vi "Acquisition Example.vi"() -> ()   [LabVIEW 2023, in "GettingStarted_Acq_148X_Host.lvlib"]
uses:
  GettingStarted_Acq_148X_Host.lvlib
  <vilib>/rvi/interface/nirviCloseFPGA/nirviCloseFPGA.xnode
  <instrlib>/FlexRIO/API/Host/v1/NI FlexRIO API v1.lvlib
  Common/GettingStarted_Common_148X_Host.lvlib
  <vilib>/vision/Image Controls.llb/IMAQ Image.ctl
  Common/Types/Packet Table.ctl
  <vilib>/Utility/miscctls.llb/LVRowAndColumnUnsignedTypeDef.ctl
  <vilib>/FPGAPlugInAG/Dynamic/niLvFpga_Close_Dynamic.vi
  <instrlib>/FlexRIO/API/Host/v1/NI FlexRIO/API/Wait for PoC Safe to Disconnect Channels Array.vi
  <instrlib>/FlexRIO/CSI-2/v2/Common/Types/LLP Data Type.ctl
  <instrlib>/FlexRIO/CSI-2/v2/Common/NI CSI-2 API Common v2.lvlib
  <vilib>/userDefined/Silver/nirio_resource_slv.ctl
  Types/CSI-2 Data Source.ctl
  Common/Types/Serial Channel Configuration.ctl
  Common/Types/RAW Interpretation for Display.ctl
  <instrlib>/FlexRIO/CSI-2/v2/FPGA/Types/Timestamp ID.ctl
  <instrlib>/FlexRIO/CSI-2/v2/FPGA/NI CSI-2 API FPGA v2.lvlib
  Common/Types/GPIO Filter.ctl
  FPGA/Common/Types/SerDes Identifier.ctl
  FPGA/Common/GettingStarted_Common_148X_FPGA.lvlib
  <instrlib>/FlexRIO/CSI-2/v2/FPGA/Types/GPIO Bank.ctl
  <instrlib>/FlexRIO/CSI-2/v2/FPGA/Types/Display Parameters.ctl
panel:
  out "Acquisition Stopped":bool
  in  "Configuration":T1(tab)
  in  "Logged Packets to Display":i64=1400
  in  "Log Packets to Disk":bool
  in  "Bitfile Path":path
  in  "TDMS File Directory":path
  in  "RIO Device":T2
  in  "Display Acquired Images":bool=TRUE
  in  "Log I2C to Disk":bool
  in  "Log GPIO to Disk":bool
  in  "Channel Configurations":T3[](array[typedef])=[{"Serial Channel"="SI0", "FPGA Display Parameters"={"virtual channel"=0.0, "payload data type"=enum."RAW 12", "frame skip count"=0, "line skip count"=0, "pixel skip count"=0.0}, "RAW Display Parameters"={"Interpretation"=enum."Bayer", "Bayer Parameters"={"Pattern"=3, "Algorithm"=0, "Red Gain"=1.0, "Green Gain"=1.0, "Blue Gain"=1.0}}}] {"RAW Display Parameters"."Bayer Parameters"."Blue Gain" min=0.0 max=3.99 step=0.1 format="%_4g"; "RAW Display Parameters"."Bayer Parameters"."Green Gain" min=0.0 max=3.99 step=0.1 format="%_4g"; "RAW Display Parameters"."Bayer Parameters"."Red Gain" min=0.0 max=3.99 step=0.1 format="%_4g"; "RAW Display Parameters"."Bayer Parameters"."Algorithm" items=["Bilinear", "VNG"]; "RAW Display Parameters"."Bayer Parameters"."Pattern" items=["GB", "GR", "BG", "RG"]}
  in  "CSI-2 Data Source":T7=1 items=["Raw", "Corrected"]
  in  "Configuration Script":path
  in  "Acquisition Duration (s)":dbl=1.0 format="%#_13g"
  in  "Continuous Acquisition":bool=TRUE
  in  "Data Type Filter":T5[](array[typedef])
  in  "Virtual Channel Filter":fxp<+,4,4>[](array[numeric])
  in  "Invert Data Type Filter":bool
  in  "Invert Virtual Channel Filter":bool
  in  "Enable First and Last Packet Select":bool=TRUE
  in  "Stop Timeout (s)":dbl=1.0
  in  "First Packet Data Type Select":T5
  in  "Last Packet Data Type Select":T5=enum."Frame End"
  in  "Serial Input Active Lane Count":i32(ring)=4 items=["1 Lane"=1, "2 Lanes"=2, "4 Lanes"=4]
  in  "Reference Clock Frequency (Hz)":dbl=25000000.0 format="%#_6p"
  in  "Power Over Coax Source":i32(ring) items=["None", "Internal", "Auxiliary"]
  in  "timestamp filter":T8[](array[typedef])
  in  "GPIO to Display":T9[](array[typedef])
  in  "GPIO Bank Select":T10
  in  "Write GPIO":bool
  in  "GPIO Bank Write":T11
  out "GPIO Bank Read":T11
  out "Acquisition Duration (s)":dbl format="%.1f"
  out "Acquisition In Progress":bool
  out "Power Over Coax Voltage (V)":dbl[](array[numeric]) format="%#.2pV"
  out "Power Over Coax Current (A)":dbl[](array[numeric]) format="%#.2pA"
  in  "Acquired Serial Input Channel Data":T12(tab)
  out "Source Rate (fps)(1st Display)":dbl
  out "Update Rate (fps)(1st Display)":dbl
  in  "Serial Channel (1st Display)":fxp<+,3,3>
  out "1st channel display":T13(plugin-control)
  out "Source Rate (fps)(2nd Display)":dbl
  out "Update Rate (fps)(2nd Display)":dbl
  out "2nd channel display":T13(plugin-control)
  in  "Serial Channel (2nd Display)":fxp<+,3,3>
  out "Bytes Acquired (1st Channel)":i64 format="%#.6p"
  out "Acquired Packets (1st Channel)":T14
  out "Packets Logged (1st Channel)":i64
  out "Bytes Acquired (2nd Channel)":i64 format="%#.6p"
  out "Acquired Packets (2nd Channel)":T14
  out "Packets Logged (2nd Channel)":i64
  out "I2C Timestamps":T14
  out "GPIO Timestamps Waveform":digitalwaveform[](graph)
  out "Error Parsing GPIO Timestamps":bool
  out "Power Over Coax Source In Range":bool[](array[boolean])
  in  "Stop Acquisition":bool
  out "Error Out":errorcluster
  # "Overview: Configure an acquisition for a CSI-2 sensor and transfer the acquired data and timestamps to disk.  \nInstructions: Visit https://ni.com/r/automotive-camera-module-ref for tutorials and reference material on using this example with the PXIe-148X."
  # "Configuration Settings"
  # "Data Output"
  # "Resource Configuration"
  # "Data Output Configuration"
  # "Channel Configuration"
  # "Acquisition Configuration"
  # "First and Last Packet Select Configuration"
  # "Packet Filter Configuration"
  # "Power Over Coax Configuration"
  # "Clocking Configuration"
  # "I2C Timestamp Configuration"
  # "The timestamp filters listed correspond to the I2C traffic for a specific serial channel:\n\nUser24 = SI0\nUser25 = SI1\nUser26 = SI2\nUser27 = SI3\nUser28 = SI4\nUser29 = SI5\nUser30 = SI6\nUser31 = SI7"
  # "GPIO Configuration"
  # "* For additional packet viewing capability, use GettingStarted_Common_148X_Host.lvlib->TDMS File Viewer.vi"
  # "* For additional packet viewing capability, use GettingStarted_Common_148X_Host.lvlib->TDMS File Viewer.vi"
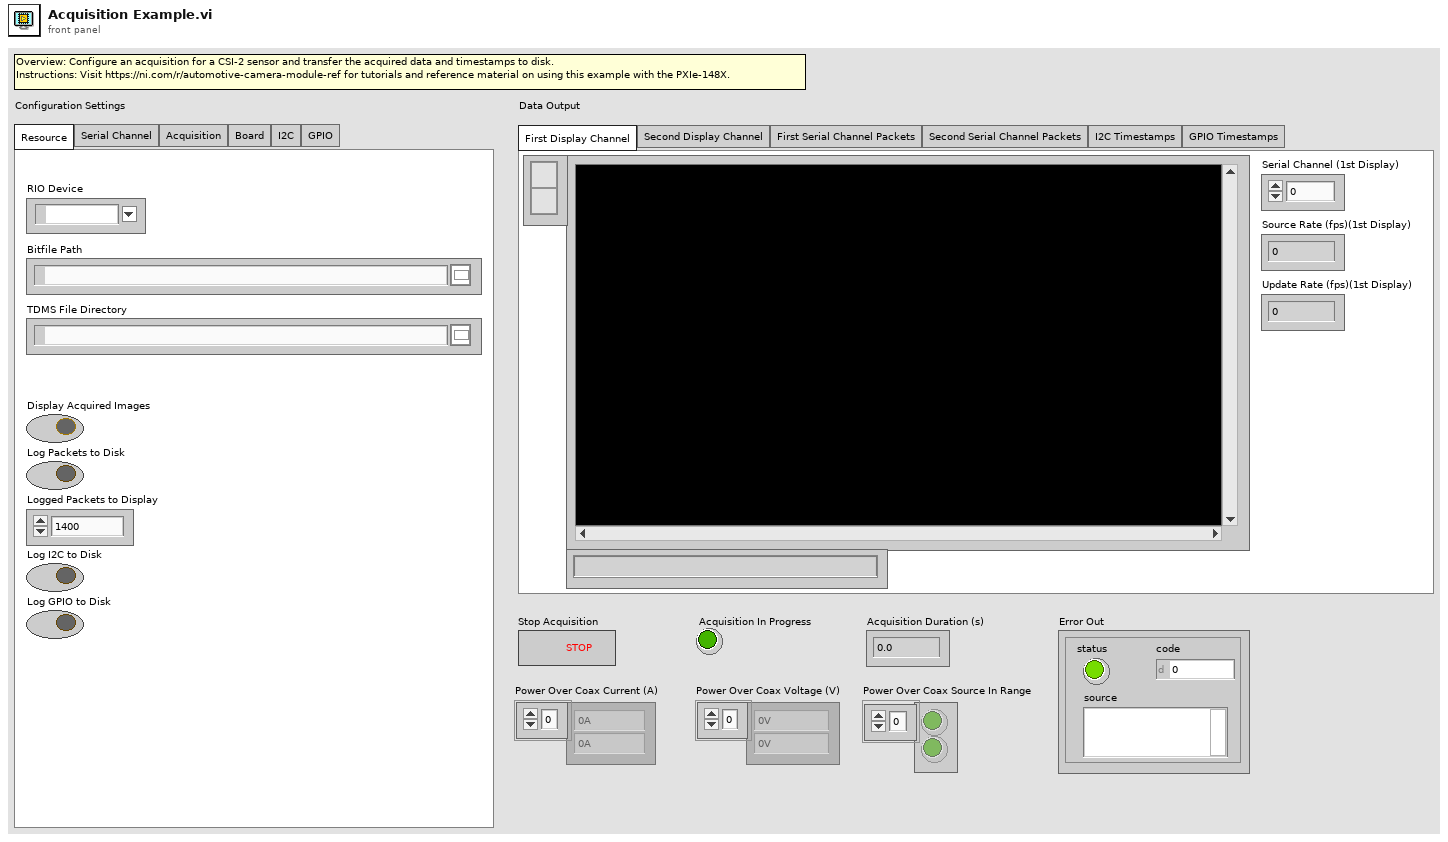
[diagram p1: front panel]
types:
  T1 = enum32{"Resource", "Serial Channel", "Acquisition", "Board", "I2C", "GPIO"}
  T2 = typedef "nirio_resource_slv.ctl" = tag
  T3 = typedef "GettingStarted_Common_148X_Host.lvlib/Serial Channel Configuration.ctl" = cluster{"Serial Channel":string, "FPGA Display Parameters":T4, "RAW Display Parameters":cluster{"Interpretation":T6, "Bayer Parameters":cluster{"Pattern":i32, "Algorithm":i32, "Red Gain":dbl, "Green Gain":dbl, "Blue Gain":dbl}}}
  T4 = typedef "NI CSI-2 API FPGA v2.lvlib/Display Parameters.ctl" = cluster{"virtual channel":fxp<+,4,4>, "payload data type":T5, "frame skip count":u16, "line skip count":u8, "pixel skip count":fxp<+,5,5>}
  T5 = typedef "NI CSI-2 API Common v2.lvlib/LLP Data Type.ctl" = enum8{"Frame Start", "Frame End", "Line Start", "Line End", "End of Transmission", "Reserved 0", "Reserved 1", "Reserved 2", "Generic Short Packet 1", "Generic Short Packet 2", "Generic Short Packet 3", "Generic Short Packet 4", "Generic Short Packet 5", "Generic Short Packet 6", "Generic Short Packet 7", "Generic Short Packet 8", "Null", "Blanking Data", "Embedded 8-bit non Image Data", "Generic Long Packet 1", "Generic Long Packet 2", "Generic Long Packet 3", "Generic Long Packet 4", "Reserved 3", "YUV420 8-bit", "YUV420 10-bit", "Legacy YUV420 8-bit", "Reserved 4", "YUV420 8-bit Chroma Shifted", "YUV420 10-bit Chroma Shifted", "YUV422 8-bit", "YUV422 10-bit", "RGB444", "RGB555", "RGB565", "RGB666", "RGB888", "Reserved 5", "Reserved 6", "RAW 24", "RAW 6", "RAW 7", "RAW 8", "RAW 10", "RAW 12", "RAW 14", "RAW 16", "RAW 20", "User Defined 8-bit Data 1", "User Defined 8-bit Data 2", "User Defined 8-bit Data 3", "User Defined 8-bit Data 4", "User Defined 8-bit Data 5", "User Defined 8-bit Data 6", "User Defined 8-bit Data 7", "User Defined 8-bit Data 8", "USL Command", "Reserved 7", "Reserved 8", "Reserved 9", "Reserved 10", "Reserved 11", "Reserved 12", "LRTE EPD Spacer"}
  T6 = typedef "GettingStarted_Common_148X_Host.lvlib/RAW Interpretation for Display.ctl" = enum16{"Grayscale", "Bayer", "RGB", "YUV422", "YUV420", "Legacy YUV420"}
  T7 = typedef "GettingStarted_Acq_148X_Host.lvlib/CSI-2 Data Source.ctl" = u16
  T8 = typedef "NI CSI-2 API FPGA v2.lvlib/Timestamp ID.ctl" = enum8{"SI0 LLP", "SI1 LLP", "SI2 LLP", "SI3 LLP", "SI4 LLP", "SI5 LLP", "SI6 LLP", "SI7 LLP", "SO0 LLP", "SO1 LLP", "SO2 LLP", "SO3 LLP", "SO4 LLP", "SO5 LLP", "SO6 LLP", "SO7 LLP", "Ser0 GPIO Bank", "Ser1 GPIO Bank", "Ser2 GPIO Bank", "Ser3 GPIO Bank", "Ser4 GPIO Bank", "Ser5 GPIO Bank", "Ser6 GPIO Bank", "Ser7 GPIO Bank", "Des0 GPIO Bank", "Des1 GPIO Bank", "Des2 GPIO Bank", "Des3 GPIO Bank", "Des4 GPIO Bank", "Des5 GPIO Bank", "Des6 GPIO Bank", "Des7 GPIO Bank", "User0", "User1", "User2", "User3", "User4", "User5", "User6", "User7", "User8", "User9", "User10", "User11", "User12", "User13", "User14", "User15", "User16", "User17", "User18", "User19", "User20", "User21", "User22", "User23", "User24", "User25", "User26", "User27", "User28", "User29", "User30", "User31"}
  T9 = typedef "GettingStarted_Common_148X_Host.lvlib/GPIO Filter.ctl" = cluster{"GPIO Bank":T8, "GPIO Number":i32}
  T10 = typedef "GettingStarted_Common_148X_FPGA.lvlib/SerDes Identifier.ctl" = enum8{"None", "SI 0 Deserializer", "SI 1 Deserializer", "SI 2 Deserializer", "SI 3 Deserializer", "SI 4 Deserializer", "SI 5 Deserializer", "SI 6 Deserializer", "SI 7 Deserializer", "SO 0 Serializer", "SO 1 Serializer", "SO 2 Serializer", "SO 3 Serializer", "SO 4 Serializer", "SO 5 Serializer", "SO 6 Serializer", "SO 7 Serializer", "SI 0 SI 1 Deserializer", "SI 2 SI 3 Deserializer", "SI 4 SI 5 Deserializer", "SI 6 SI 7 Deserializer"}
  T11 = typedef "NI CSI-2 API FPGA v2.lvlib/GPIO Bank.ctl" = cluster{"GPIO 0":bool, "GPIO 1":bool, "GPIO 2":bool, "GPIO 3":bool, "GPIO 4":bool, "GPIO 5":bool, "GPIO 6":bool, "GPIO 7":bool, "GPIO 8":bool, "GPIO 9":bool, "GPIO 10":bool}
  T12 = enum32{"First Display Channel", "Second Display Channel", "First Serial Channel Packets", "Second Serial Channel Packets", "I2C Timestamps", "GPIO Timestamps"}
  T13 = typedef "IMAQ Image.ctl" = refnum<image>
  T14 = typedef "GettingStarted_Common_148X_Host.lvlib/Packet Table.ctl" = string[][]
  T15 = typedef "LVRowAndColumnUnsignedTypeDef.ctl" = cluster{"Row":u32, "Column":u32}
  T16 = typedef "GettingStarted_Common_148X_Host.lvlib/Serial Channel Display Parameters.ctl" = cluster{"images":cluster{"grayscale":T13, "color":T13}, "RAW parameters":cluster{"interpretation":T6, "bayer parameters":cluster{"pattern":i32, "algorithm":i32, "red gain":dbl, "green gain":dbl, "blue gain":dbl}}}
  T17 = cluster{"Source Rate (fps)(1st Display)":refnum<vi>, "Update Rate (fps)(1st Display)":refnum<vi>}
  T18 = cluster{"Source Rate (fps)(2nd Display)":refnum<vi>, "Update Rate (fps)(2nd Display)":refnum<vi>}
  T19 = cluster{"Source Rate (fps)(2nd Display)":refnum<vi>, "Update Rate (fps)(2nd Display)":refnum<vi>}[]
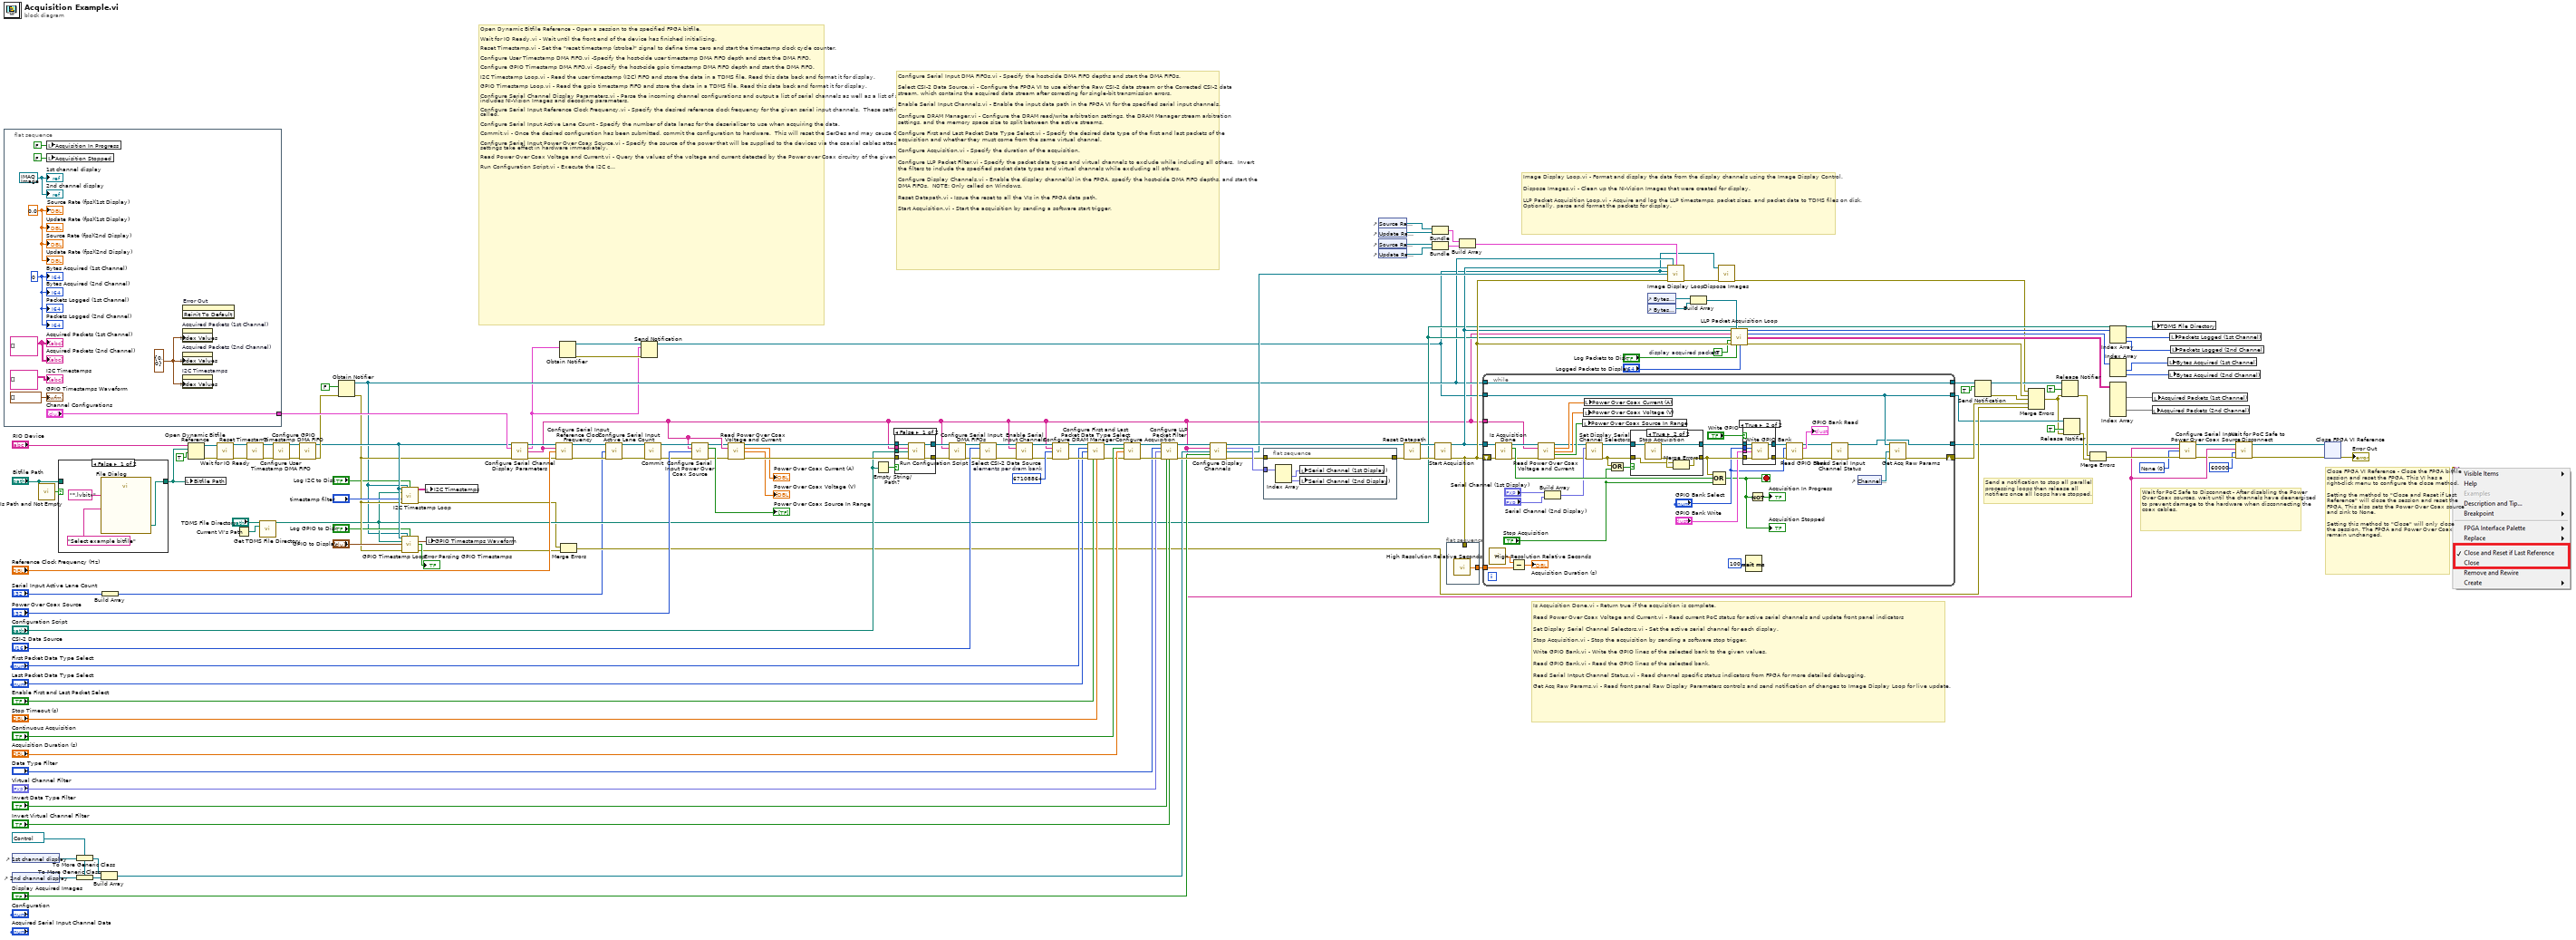
[diagram p0: block diagram]
diagram:
  w4 = 0 items=["None", "Internal", "Auxiliary"] ("power over coax source")
  w31 = TRUE  # display acquired packets
  w82 = refnum<vi> refnum ("image display reference")
  w148 = u32 67108864  # elements per dram bank
  # "Wait for PoC Safe to Disconnect - After disabling the Power Over Coax sources, wait until the channels have deenergized to prevent damage to the hardware when disconnecting the coax cables."
  # "Send a notification to stop all parallel processing loops then release all notifiers once all loops have stopped."
  # "Image Display Loop.vi - Format and display the data from the display channels using the Image Display Control.   \n\nDispose Images.vi - Clean up the NI-Vision Images that were created for display.\n\nLLP Packet Acquisition Loop.vi - Acquire and log the LLP timestamps, packet sizes, and packet data to TDMS files on disk.  Optionally, parse and format the packets for display."
  # "Configure Serial Input DMA FIFOs.vi - Specify the host-side DMA FIFO depths and start the DMA FIFOs.\n\nSelect CSI-2 Data Source.vi - Configure the FPGA VI to use either the Raw CSI-2 data stream or the Corrected CSI-2 data stream, which contains the acquired data stream after correcting for single-bit transmission errors.\n\nEnable Serial Input Channels.vi - Enable the input data path in the FPGA VI for the specified serial input channels.\n\nConfigure DRAM Manager.vi - Configure the DRAM read/write arbitration settings, the DRAM Manager stream arbitration settings, and the memory space size to split between the active streams.\n\nConfigure First and Last Packet Data Type Select.vi - Specify the desired data type of the first and last packets of the acquisition and whether they must come from the same virtual channel.\n\nConfigure Acquisition.vi - Specify the duration of the acquisition.\n\nConfigure LLP Packet Filter.vi - Specify the packet data types and virtual channels to exclude while including all others.  Invert the filters to include the specified packet data types and virtual channels while excluding all others.\n\nConfigure Display Channels.vi - Enable the display channel(s) in the FPGA, specify the host-side DMA FIFO depths, and start the DMA FIFOs.  NOTE: Only called on Windows. \n\nReset Datapath.vi - Issue the reset to all the VIs in the FPGA data path.\n\nStart Acquisition.vi - Start the acquisition by sending a software start trigger."
  # "Close FPGA VI Reference - Close the FPGA bitfile session and reset the FPGA. This VI has a right-click menu to configure the close method. \n\nSetting the method to \"Close and Reset if Last Reference\" will close the session and reset the FPGA. This also sets the Power Over Coax source and sink to None.\n\nSetting this method to \"Close\" will only close the session. The FPGA and Power Over Coax remain unchanged."
  # "Open Dynamic Bitfile Reference - Open a session to the specified FPGA bitfile.\n\nWait for IO Ready.vi - Wait until the front end of the device has finished initializing.\n\nReset Timestamp.vi - Set the \"reset timestamp (strobe)\" signal to define time zero and start the timestamp clock cycle counter.\n\nConfigure User Timestamp DMA FIFO.vi -Specify the host-side user timestamp DMA FIFO depth and start the DMA FIFO.\n\nConfigure GPIO Timestamp DMA FIFO.vi -Specify the host-side gpio timestamp DMA FIFO depth and start the DMA FIFO.\n\nI2C Timestamp Loop.vi - Read the user timestamp (I2C) FIFO and store the data in a TDMS file. Read this data back and format it for display.\n\nGPIO Timestamp Loop.vi - Read the gpio timestamp FIFO and store the data in a TDMS file. Read this data back and format it for display.\n\nConfigure Serial Channel Display Parameters.vi - Parse the incoming channel configurations and output a list of serial channels as well as a list of serial channel display parameters, which includes NI-Vision Images and decoding parameters.\n\nConfigure Serial Input Reference Clock Frequency.vi - Specify the desired reference clock frequency for the given serial input channels.  These settings do not take effect until Commit.vi is called.\n\nConfigure Serial Input Active Lane Count - Specify the number of data lanes for the deserializer to use when acquiring the data. \n\nCommit.vi - Once the desired configuration has been submitted, commit the configuration to hardware.  This will reset the SerDes and may cause GPIO lines to toggle. \n\nConfigure Serial Input Power Over Coax Source.vi - Specify the source of the power that will be supplied to the devices via the coaxial cables attached to the given serial input channels.  These settings take effect in hardware immediately.\n\nRead Power Over Coax Voltage and Current.vi - Query the values of the voltage and current detected by the Power over Coax circuitry of the given serial channels.\n\nRun Configuration Script.vi - Execute the I2C commands in the specified script file for the given serial channels.  The script is used to configure the serializer, deserializer, or other I2C slave device, such as the image sensor."
  # "Is Acquisition Done.vi - Return true if the acquisition is complete.\n\nRead Power Over Coax Voltage and Current.vi - Read current PoC status for active serial channels and update front panel indicators \n\nSet Display Serial Channel Selectors.vi - Set the active serial channel for each display.\n\nStop Acquisition.vi - Stop the acquisition by sending a software stop trigger.\n\nWrite GPIO Bank.vi - Write the GPIO lines of the selected bank to the given values.\n\nRead GPIO Bank.vi - Read the GPIO lines of the selected bank.\n\nRead Serial Intput Channel Status.vi - Read channel specific status indicators from FPGA for more detailed debugging.\n\nGet Acq Raw Params.vi - Read front panel Raw Display Parameters controls and send notification of changes to Image Display Loop for live update."
  n1 = flat-sequence {
    tunnel: ["Channel Configurations"] -> w96
    frame #0 {
      w149 = T15 {"Row"=0, "Column"=0} ("Index Values")
      w156 = T14 [] ("Acquired Packets (1st Channel)")
      w152 = 0 ("Number of Packets Acquired (1st Channel)")
      w155 = 0.0 ("display fps (2nd display)")
      w158 = T13 refnum ("first channel display")
      n2 = local write "Acquisition In Progress"(FALSE ("Acquisition In Progress")) -> ()
      n3 = local write "Acquisition Stopped"(FALSE ("Acquisition Stopped")) -> ()
      n4 = property on="Acquired Packets (1st Channel)" class="Tbl (strict)"("Index Values"=w149) -> ()  [unwired: 2 in, 2 out]
      n5 = property on="Acquired Packets (2nd Channel)" class="Tbl (strict)"("Index Values"=w149) -> ()  [unwired: 2 in, 2 out]
      n6 = property on="I2C Timestamps" class="Tbl (strict)"("Index Values"=w149) -> ()  [unwired: 2 in, 2 out]
      n7 = invoke on="Error Out" class="Clust (strict)" method="Reinit To Default"() -> ()  [unwired: 3 in, 3 out]
      "1st channel display" <- w158
      "2nd channel display" <- w158
      "Update Rate (fps)(1st Display)" <- w155
      "Update Rate (fps)(2nd Display)" <- w155
      "Acquired Packets (1st Channel)" <- w156
      "Packets Logged (1st Channel)" <- w152
      "Acquired Packets (2nd Channel)" <- w156
      "Packets Logged (2nd Channel)" <- w152
      "Source Rate (fps)(1st Display)" <- w155
      "Source Rate (fps)(2nd Display)" <- w155
      "GPIO Timestamps Waveform" <- digitalwaveform[] [] ("GPIO Timestamps Waveform")
      "I2C Timestamps" <- T14 [] ("I2C Timestamps 2")
      "Bytes Acquired (1st Channel)" <- w152
      "Bytes Acquired (2nd Channel)" <- w152
    }
  }
  n8 = control-ref of="1st channel display"() -> (w93:refnum<vi>)
  n9 = control-ref of="2nd channel display"() -> (w91:refnum<vi>)
  n10 = call <vilib>:"Is Path and Not Empty.vi"("path"="Bitfile Path") -> ("Is Path and Not Empty?"=w130:bool)  [unwired: 4 in]
  n11 = case shown="False" w130 {
    tunnel: "Bitfile Path" -> [_ w162]
    tunnel: [w160 w162] -> w129
    frame False {
      n12 = call "File Dialog"("prompt"="Select example bitfile", "pattern (all files)"="*.lvbitx") -> ("selected path"=w160:path)  [unwired: 10 in, 3 out]
    }
    frame True {
    }
  }
  n13 = To More Generic Class(target class=w82, reference=w93) -> (generic class reference=w92:refnum<vi>)
  n14 = To More Generic Class(target class=w82, reference=w91) -> (generic class reference=w90:refnum<vi>)
  n15 = Build Array(w92, w90) -> (w88:refnum<vi>[])
  n16 = Build Array("Serial Input Active Lane Count") -> (w22:i32[])
  n17 = local write "Bitfile Path"(w129) -> ()
  n18 = Open Dynamic Bitfile Reference(0:"RIO Device", 1:w129, 2:TRUE ("Run When Loaded")) -> (5:w127:refnum<k20>, 8:w128:errorcluster)  [unwired: 2 in]
  n19 = call <instrlib>:"Wait for IO Ready.vi"("fpga interface in"=w127, "error in"=w128) -> ("fpga interface out"=w60:refnum<k20>, "error out"=w61:errorcluster)  [unwired: 10 in, 2 out]
  n20 = Current VI's Path() -> (path=w100:path)
  n21 = call "Reset Timestamp.vi"("fpga interface in"=w60, "error in (no error)"=w61) -> ("fpga interface out"=w50:refnum<k20>, "error out"=w49:errorcluster)  [unwired: 12 in]
  n22 = call "Get TDMS File Directory.vi"("tdms file directory in"="TDMS File Directory", "calling vi path"=w100) -> ("tdms file directory out"=w35:path)  [unwired: 13 in]
  n23 = call "Configure User Timestamp DMA FIFO.vi"("fpga interface in"=w50, "error in (no error)"=w49) -> ("fpga interface out"=w48:refnum<k20>, "error out"=w47:errorcluster)  [unwired: 12 in]
  n24 = call "Configure GPIO Timestamp DMA FIFO.vi"("fpga interface in"=w48, "error in (no error)"=w47) -> ("fpga interface out"=w44:refnum<k20>, "error out"=w46:errorcluster)  [unwired: 12 in]
  n25 = Obtain Notifier(notification data type=FALSE ("result"), error in (no error)=w46) -> (notifier out=w21:refnum<notifier>, error out=w38:errorcluster)  [unwired: 2 in, 1 out]
  n26 = call "I2C Timestamp Loop.vi"("fpga interface in"=w44, "'stop' notifier"=w21, "log i2c to disk"="Log I2C to Disk", "tdms file directory"=w35, "timestamp filter"="timestamp filter", "error in (no error)"=w38) -> ("i2c data"=w43:string[][], "error out"=w33:errorcluster)  [unwired: 8 in]
  n27 = call "GPIO Timestamp Loop.vi"("fpga interface in"=w44, "'stop' notifier"=w21, "log gpio to disk"="Log GPIO to Disk", "tdms file directory"=w35, "gpio to display"="GPIO to Display", "error in (no error)"=w38) -> ("gpio timestamps waveform"=w42:digitalwaveform[], "error parsing gpio timestamps"=→"Error Parsing GPIO Timestamps":bool, "error out"=w32:errorcluster)  [unwired: 7 in]
  n28 = local write "I2C Timestamps"(w43) -> ()
  n29 = local write "GPIO Timestamps Waveform"(w42) -> ()
  n30 = call "Configure Serial Channel Display Parameters.vi"("fpga interface in"=w44, "serial channel configurations"=w96, "error in (no error)"=w38) -> ("fpga interface out"=w95:refnum<k20>, "serial channel display parameters"=w18:T16[], "serial channels"=w7:string[], "error out"=w94:errorcluster)  [unwired: 9 in]
  n31 = call "Configure Serial Input Reference Clock Frequency.vi"("fpga interface in"=w95, "serial input channels"=w7, "serial input reference clock frequency (Hz)"="Reference Clock Frequency (Hz)", "error in (no error)"=w94) -> ("fpga interface out"=w27:refnum<k20>, "error out"=w26:errorcluster)  [unwired: 10 in]
  n32 = Obtain Notifier(notification data type=w18) -> (notifier out=w20:refnum<notifier>, error out=w19:errorcluster)  [unwired: 3 in, 1 out]
  n33 = Merge Errors(w33, w32) -> (w28:errorcluster)
  n34 = call "Configure Serial Input Active Lane Count.vi"("fpga interface in"=w27, "serial input active lane counts"=w22, "error in (no error)"=w26) -> ("fpga interface out"=w25:refnum<k20>, "error out"=w24:errorcluster)  [unwired: 11 in]
  n35 = Send Notification(notification=w18, notifier=w20, error in (no error)=w19) -> (notifier out=w17:refnum<notifier>)  [unwired: 1 out]
  n36 = call <instrlib>:"Commit.vi"("fpga interface in"=w25, "error in"=w24) -> ("fpga interface out"=w134:refnum<k20>, "error out"=w135:errorcluster)  [unwired: 12 in]
  n37 = call "Configure Serial Input Power Over Coax Source.vi"("fpga interface in"=w134, "serial input channels"=w7, "power over coax source"="Power Over Coax Source", "error in (no error)"=w135) -> ("fpga interface out"=w5:refnum<k20>, "power over coax source in range"=→"Power Over Coax Source In Range":bool[], "error out"=w6:errorcluster)  [unwired: 9 in]
  n38 = call "Read Power Over Coax Voltage and Current.vi"("fpga interface in"=w5, "serial channels"=w7, "error in (no error)"=w6) -> ("fpga interface out"=w124:refnum<k20>, "current (A)"=→"Power Over Coax Current (A)":dbl[], "voltage (V)"=→"Power Over Coax Voltage (V)":dbl[], "error out"=w125:errorcluster)  [unwired: 8 in, 1 out]
  n39 = Empty String/Path?(string/path="Configuration Script") -> (empty?=w63:bool)
  n40 = case shown="False" w63 {
    tunnel: [w168 w169] -> w146
    tunnel: [w167 w170] -> w138
    tunnel: w125 -> [w166 w169]
    tunnel: w124 -> [w165 w170]
    tunnel: w7 -> [w164 _]
    tunnel: "Configuration Script" -> [w163 _]
    frame False {
      n41 = call "Run Configuration Script.vi"("fpga interface in"=w165, "serial channels"=w164, "configuration script"=w163, "error in (no error)"=w166) -> ("fpga interface out"=w167:refnum<k20>, "error out"=w168:errorcluster)  [unwired: 10 in]
    }
    frame True {
    }
  }
  n42 = call "Configure Serial Input DMA FIFOs.vi"("fpga interface in"=w138, "serial channels"=w7, "error in (no error)"=w146) -> ("fpga interface out"=w116:refnum<k20>, "error out"=w113:errorcluster)  [unwired: 11 in]
  n43 = call "Select CSI-2 Data Source.vi"("fpga interface in"=w116, "csi-2 data source"="CSI-2 Data Source", "error in (no error)"=w113) -> ("fpga interface out"=w115:refnum<k20>, "error out"=w114:errorcluster)  [unwired: 11 in]
  n44 = call "Enable Serial Input Channels.vi"("fpga interface in"=w115, "serial input channels"=w7, "error in (no error)"=w114) -> ("fpga interface out"=w137:refnum<k20>, "error out"=w147:errorcluster)  [unwired: 11 in]
  n45 = call "Configure DRAM Manager.vi"("fpga interface in"=w137, "serial channels"=w7, "elements per dram bank"=w148, "error in (no error)"=w147) -> ("fpga interface out"=w109:refnum<k20>, "error out"=w112:errorcluster)  [unwired: 10 in]
  n46 = call "Configure First and Last Packet Data Type Select.vi"("fpga interface in"=w109, "first packet data type select"="First Packet Data Type Select", "last packet data type select"="Last Packet Data Type Select", "error in (no error)"=w112, "enable first and last packet select"="Enable First and Last Packet Select", "stop timeout (s)"="Stop Timeout (s)") -> ("fpga interface out"=w110:refnum<k20>, "error out"=w111:errorcluster)  [unwired: 8 in]
  n47 = call "Configure Acquisition.vi"("fpga interface in"=w110, "continuous acquisition (T)"="Continuous Acquisition", "acquisition duration (s)"="Acquisition Duration (s)", "error in (no error)"=w111) -> ("fpga interface out"=w143:refnum<k20>, "error out"=w144:errorcluster)  [unwired: 10 in]
  n48 = call "Configure LLP Packet Filter.vi"("fpga interface in"=w143, "data type filter"="Data Type Filter", "virtual channel filter"="Virtual Channel Filter", "error in (no error)"=w144, "invert data type filter"="Invert Data Type Filter", "invert virtual channel filter"="Invert Virtual Channel Filter") -> ("fpga interface out"=w97:refnum<k20>, "error out"=w89:errorcluster)  [unwired: 8 in]
  n49 = call "Configure Display Channels.vi"("fpga interface in"=w97, "serial channels"=w7, "display references in"=w88, "enable image display"="Display Acquired Images", "error in (no error)"=w89) -> ("fpga interface out"=w87:refnum<k20>, "display serial channels"=w86:fxp<+,3,3>[], "display references out"=w83:refnum<vi>[], "error out"=w85:errorcluster)  [unwired: 7 in]
  n50 = flat-sequence {
    tunnel: w86 -> [w172]
    tunnel: w85 -> [w171]
    tunnel: [w171] -> w84
    frame #0 {
      n51 = Index Array(array=w172) -> (element #1=w174:fxp<+,3,3>, element #2=w173:fxp<+,3,3>)  [unwired: 2 in]
      n52 = local write "Serial Channel (1st Display)"(w174) -> ()
      n53 = local write "Serial Channel (2nd Display)"(w173) -> ()
    }
  }
  n54 = control-ref of="Source Rate (fps)(1st Display)"() -> (w75:refnum<vi>)
  n55 = control-ref of="Update Rate (fps)(1st Display)"() -> (w76:refnum<vi>)
  n56 = control-ref of="Source Rate (fps)(2nd Display)"() -> (w74:refnum<vi>)
  n57 = control-ref of="Update Rate (fps)(2nd Display)"() -> (w73:refnum<vi>)
  n58 = call "Reset Datapath.vi"("fpga interface in"=w87, "error in (no error)"=w84) -> ("fpga interface out"=w145:refnum<k20>, "error out"=w45:errorcluster)  [unwired: 12 in]
  n59 = Bundle("Source Rate (fps)(1st Display)"=w75, "Update Rate (fps)(1st Display)"=w76) -> (w72:T17)  [unwired: 1 in]
  n60 = Bundle("Source Rate (fps)(2nd Display)"=w74, "Update Rate (fps)(2nd Display)"=w73) -> (w71:T18)  [unwired: 1 in]
  n61 = call "Start Acquisition.vi"("fpga interface in"=w145, "error in (no error)"=w45) -> ("fpga interface out"=w58:refnum<k20>, "error out"=w59:errorcluster)  [unwired: 12 in]
  n62 = flat-sequence {
    tunnel: [w175] -> w102
    tunnel: w59 -> [_]
    frame #0 {
      n63 = call <vilib>:"High Resolution Relative Seconds.vi"() -> ("relative seconds"=w175:dbl)
    }
  }
  n64 = Build Array(w72, w71) -> (w70:T19)
  n65 = while {
    shift-right: [w182] -> w29
    shift-left: w59 -> [w184]
    tunnel: w58 -> [w198]
    tunnel: w7 -> [w210]
    tunnel: w102 -> [w205]
    tunnel: w21 -> [w183]
    tunnel: [w183] -> w55
    tunnel: w17 -> [w180]
    tunnel: [w176] -> w11
    tunnel: [w180] -> w15
    stop <- w185 stop-if-true
    n66 = call <vilib>:"High Resolution Relative Seconds.vi"() -> ("relative seconds"=w206:dbl)
    n67 = call "Is Acquisition Done.vi"("fpga interface in"=w198, "error in (no error)"=w184) -> ("fpga interface out"=w211:refnum<k20>, "acquisition done"=w215:bool, "error out"=w212:errorcluster)  [unwired: 11 in]
    n68 = Subtract(x=w206, y=w205) -> (x-y=→"Acquisition Duration (s)":dbl)
    n69 = call "Read Power Over Coax Voltage and Current.vi"("fpga interface in"=w211, "serial channels"=w210, "error in (no error)"=w212) -> ("fpga interface out"=w200:refnum<k20>, "current (A)"=w209:dbl[], "voltage (V)"=w207:dbl[], "in range"=w208:bool[], "error out"=w199:errorcluster)  [unwired: 8 in]
    n70 = Build Array("Serial Channel (1st Display)", "Serial Channel (2nd Display)") -> (w201:fxp<+,3,3>[])
    n71 = local write "Power Over Coax Source In Range"(w208) -> ()
    n72 = local write "Power Over Coax Voltage (V)"(w207) -> ()
    n73 = local write "Power Over Coax Current (A)"(w209) -> ()
    n74 = call "Set Display Serial Channel Selectors.vi"("fpga interface in"=w200, "display serial channel selectors"=w201, "error in (no error)"=w199) -> ("fpga interface out"=w195:refnum<k20>, "error out"=w197:errorcluster)  [unwired: 11 in]
    n75 = Compound Arithmetic op=OR(w197, "Stop Acquisition") -> (w196:bool)
    n76 = case shown="True" w196 {
      tunnel: [w225 w227] -> w193
      tunnel: w197 -> [w225 w226]
      tunnel: [w224 w229] -> w194
      tunnel: w195 -> [w224 w228]
      frame False {
      }
      frame True {
        n77 = call "Stop Acquisition.vi"("fpga interface in"=w228) -> ("fpga interface out"=w229:refnum<k20>, "error out"=w230:errorcluster)  [unwired: 13 in]
        n78 = Merge Errors(w226, w230) -> (w227:errorcluster)
      }
    }
    n79 = Compound Arithmetic op=OR(w193, w215, "Stop Acquisition") -> (w185:bool)
    "Acquisition Stopped" <- w185
    n80 = case shown="True" "Write GPIO" {
      tunnel: w194 -> [w217 w223]
      tunnel: w193 -> [w216 w222]
      tunnel: "GPIO Bank Write" -> [_ w221]
      tunnel: [w217 w220] -> w191
      tunnel: [w216 w219] -> w190
      tunnel: "GPIO Bank Select" -> [_ w218]
      frame False {
      }
      frame True {
        n81 = call "Write GPIO Bank.vi"("fpga interface in"=w223, "gpio bank select"=w218, "gpio bank output"=w221, "error in (no error)"=w222) -> ("fpga interface out"=w220:refnum<k20>, "error out"=w219:errorcluster)  [unwired: 10 in]
      }
    }
    n82 = Wait (ms)(milliseconds to wait=u32 100) -> ()  [unwired: 1 out]
    n83 = Not(x=w185) -> (.not. x?=→"Acquisition In Progress":bool)
    n84 = call "Read GPIO Bank.vi"("fpga interface in"=w191, "gpio bank select"="GPIO Bank Select", "error in (no error)"=w190) -> ("fpga interface out"=w177:refnum<k20>, "gpio bank output"=→"GPIO Bank Read":T11, "error out"=w179:errorcluster)  [unwired: 10 in]
    n85 = call "Read Serial Input Channel Status.vi"("fpga interface in"=w177, "error in (no error)"=w179) -> ("fpga interface out"=w176:refnum<k20>, "error out"=w178:errorcluster)  [unwired: 11 in, 1 out]
    n86 = control-ref of="Channel Configurations"() -> (w181:refnum<vi>)
    n87 = call "Get Acq Raw Params.vi"("raw display notifier"=w180, "Channel Configurations"=w181, "error in (no error)"=w178) -> ("error out"=w182:errorcluster)  [unwired: 12 in]
  }
  n88 = control-ref of="Bytes Acquired (1st Channel)"() -> (w104:refnum<vi>)
  n89 = control-ref of="Bytes Acquired (2nd Channel)"() -> (w103:refnum<vi>)
  n90 = call "Image Display Loop.vi"("fpga interface in"=w58, "'stop' notifier"=w21, "rate references"=w70, "raw display notifier"=w17, "display references"=w83, "error in (no error)"=w59) -> ("error out"=w77:errorcluster)  [unwired: 9 in]
  n91 = Build Array(w104, w103) -> (w99:refnum<vi>[])
  n92 = call "Dispose Images.vi"("raw display notifier"=w17, "error in (no error)"=w77) -> ("error out"=w34:errorcluster)  [unwired: 13 in]
  n93 = call "LLP Packet Acquisition Loop.vi"("fpga interface in"=w58, "bytes acquired references"=w99, "Serial Channels"=w7, "tdms file directory"=w35, "display acquired packets"=w31, "error in"=w59, "log to disk"="Log Packets to Disk", "num packets to read"="Logged Packets to Display") -> ("number of packets acquired"=w98:i64[], "number of bytes acquired"=w67:i64[], "display data"=w68:string[][][], "error out"=w56:errorcluster)  [unwired: 4 in]
  n94 = Send Notification(notification=TRUE, notifier=w55) -> (notifier out=w54:refnum<notifier>, error out=w53:errorcluster)  [unwired: 1 in]
  n95 = Merge Errors(w34, w56, w53, w29, w28) -> (w14:errorcluster)
  n96 = Release Notifier(notifier=w54, force destroy? (F)=TRUE, error in (no error)=w14) -> (error out=w13:errorcluster)  [unwired: 2 out]
  n97 = Release Notifier(notifier=w15, force destroy? (F)=TRUE, error in (no error)=w14) -> (error out=w12:errorcluster)  [unwired: 2 out]
  n98 = Merge Errors(w13, w12) -> (w10:errorcluster)
  n99 = Index Array(array=w98) -> (element #1=w81:i64, element #2=w80:i64)  [unwired: 2 in]
  n100 = Index Array(array=w67) -> (element #1=w66:i64, element #2=w65:i64)  [unwired: 2 in]
  n101 = Index Array(array=w68) -> (element #1=w79:string[][], element #2=w78:string[][])  [unwired: 6 in]
  n102 = local write "TDMS File Directory"(w35) -> ()
  n103 = local write "Acquired Packets (2nd Channel)"(w78) -> ()
  n104 = local write "Acquired Packets (1st Channel)"(w79) -> ()
  n105 = local write "Bytes Acquired (1st Channel)"(w66) -> ()
  n106 = local write "Bytes Acquired (2nd Channel)"(w65) -> ()
  n107 = local write "Packets Logged (1st Channel)"(w81) -> ()
  n108 = local write "Packets Logged (2nd Channel)"(w80) -> ()
  n109 = call "Configure Serial Input Power Over Coax Source.vi"("fpga interface in"=w11, "serial input channels"=w7, "power over coax source"=w4, "error in (no error)"=w10) -> ("fpga interface out"=w2:refnum<k20>, "error out"=w3:errorcluster)  [unwired: 9 in, 1 out]
  n110 = call-poly <instrlib>:"Wait for PoC Safe to Disconnect.vi"("error in"=w3, "Timeout (ms)"=60000 ("Wait for Safe to Disconnect Timeout (ms)"), "Channels"=w7, "fpga interface in"=w2) -> ("error out"=w9:errorcluster, "fpga interface out"=w8:refnum<k20>)  [unwired: 6 in]
  n111 = xnode ("Close FPGA VI Reference")("FPGA VI Reference In"=w8, "error in"=w9) -> ("error out"=→"Error Out":errorcluster)
